vi "Wait_Sec.vi"(0 "Delay Time (sec)":dbl=1.0, 1 "error out":errorcluster) -> (4 "error in":errorcluster)   [LabVIEW 2017]
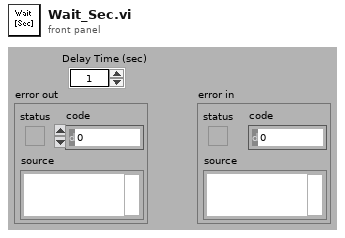
[diagram p1: front panel]
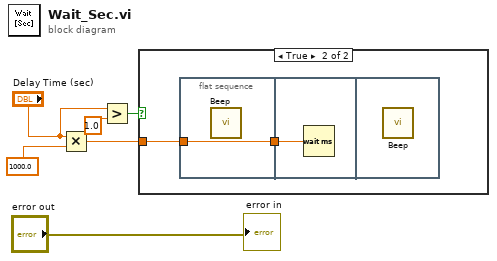
[diagram p0: block diagram]
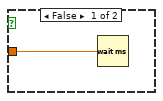
[diagram p2: hidden frame]
diagram:
  n1 = Multiply(x="Delay Time (sec)", y=1000.0) -> (x*y=w1:dbl)
  n2 = Greater?(x="Delay Time (sec)", y=1.0) -> (0:w2:bool)
  n3 = case shown="True" w2 {
    tunnel: w1 -> [w7 w8]
    frame False {
      n4 = Wait (ms)(milliseconds to wait=w7) -> ()  [unwired: 1 out]
    }
    frame True {
      n5 = flat-sequence {
        tunnel: w8 -> [w10]
        tunnel: [w10] -> w9
        tunnel: w9 -> [w11]
        frame #0 {
          n6 = call <vilib>:"Beep.vi"() -> ()  [unwired: 12 in]
        }
        frame #1 {
          n7 = Wait (ms)(milliseconds to wait=w11) -> ()  [unwired: 1 out]
        }
        frame #2 {
          n8 = call <vilib>:"Beep.vi"() -> ()  [unwired: 12 in]
        }
      }
    }
  }
  "error in" <- "error out"
